vi "test Get-Set-Get Default Word Value.vi"(8 "error in":errorcluster, 11 "TestCase in":refnum<class "Scripting.lvclass">) -> (0 "error out":errorcluster, 3 "TestCase out":refnum<class "Scripting.lvclass">)   [LabVIEW 2020, in "Scripting.lvclass"]
uses:
  Scripting.lvclass
  Scripting.lvclass/Scripting.ctl
  <vilib>/addons/_JKI Toolkits/VI Tester/TestCase.llb/TestCase.lvclass
  Scripting/Ballard/Ballard ARINC 429 Scripting.lvlib
  Scripting/ARINC 429/ARINC 429 Scripting.lvlib
  C:/Program Files (x86)/National Instruments/LabVIEW 2020/vi.lib/addons/_JKI Toolkits/VI Tester/TestCase.llb/TestCase.lvclass
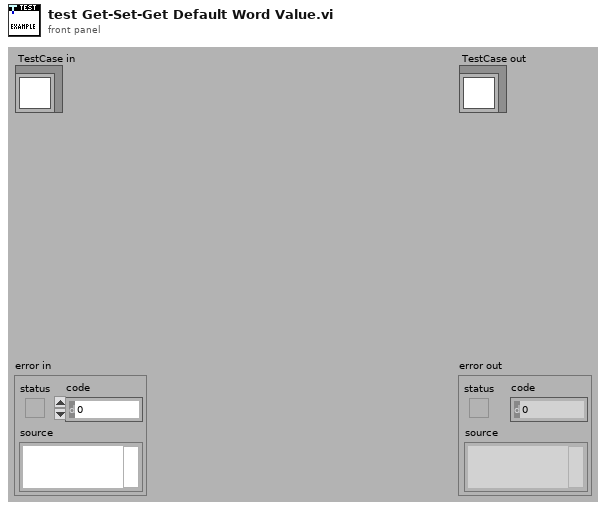
[diagram p1: front panel]
types:
  T1 = typedef "Custom Device API.lvlib/Custom Device Item Ref.ctl" = u64
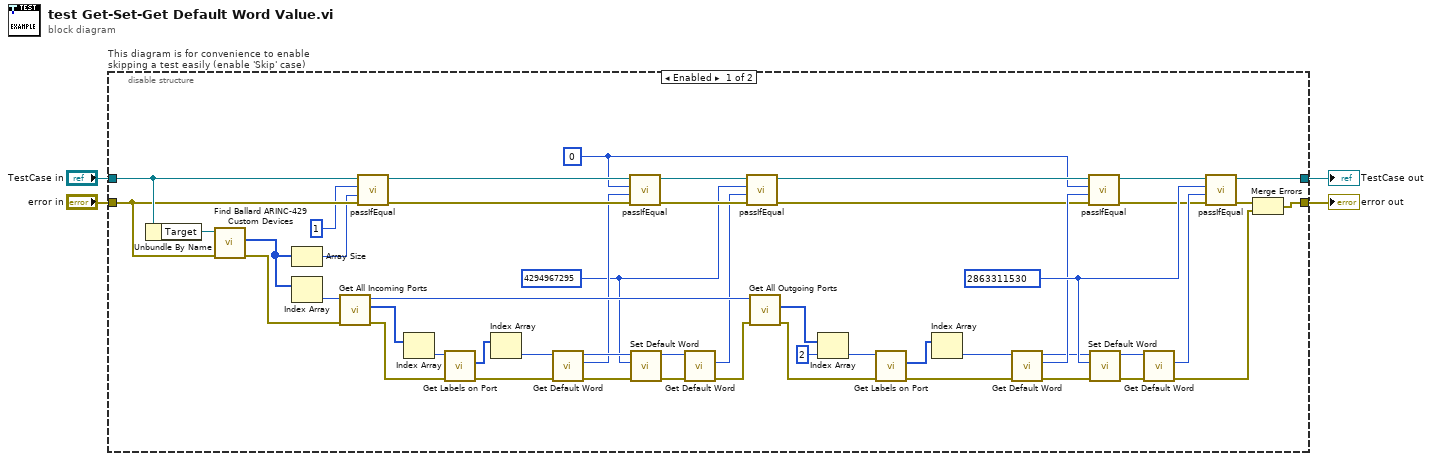
[diagram p0: block diagram]
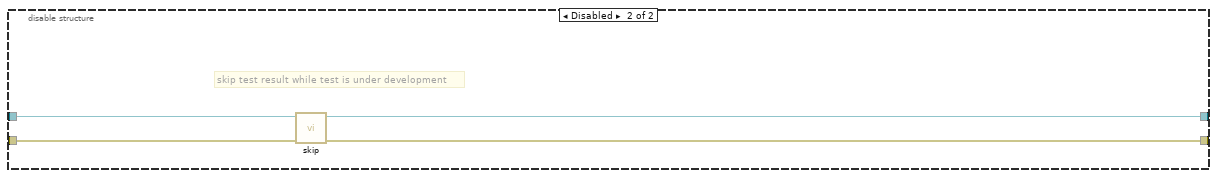
[diagram p2: hidden frame]
diagram:
  n1 = disable-structure "This diagram is for convenience to enable skipping a test easily (enable 'Skip' case)" shown="Enabled" {
    disable-tunnel: "TestCase in" -> [w52 w58]
    disable-tunnel: [w7 w56] -> w1
    disable-tunnel: [w43 w57] -> w3
    disable-tunnel: "error in" -> [w51 w55]
    frame Enabled {
      w21 = u32 2863311530 ("default word")
      w25 = u32 4294967295 ("default word")
      w6 = u32 0 ("default word")
      n2 = Unbundle By Name(w52) -> ("Target"=w54:refnum<k24>)
      n3 = call "Find Ballard ARINC-429 Custom Devices.vi"("error in"=w51, "target in"=w54) -> ("error out"=w47:errorcluster, "Ballard ARINC 429 custom devices"=w5:u64[])  [unwired: 7 in, 1 out]
      n4 = Array Size(array=w5) -> (size(s)=w49:i32)
      n5 = Index Array(array=w5) -> (element=w53:u64)  [unwired: 1 in]
      n6 = call "Get All Incoming Ports.vi"("error in"=w47, "Ballard ARINC 429 ref"=w53) -> ("error out"=w41:errorcluster, "Port refs"=w48:T1[], "Ballard ARINC 429 ref out"=w46:T1)  [unwired: 7 in]
      n7 = call-dynamic "passIfEqual.vi"("error in (no error)"=w51, "y"=w49, "x"=1 ("size(s)"), "TestCase in"=w52) -> ("error out"=w29:errorcluster, "TestCase out"=w30:refnum<class "Scripting.lvclass">)  [unwired: 6 in]
      n8 = Index Array(array=w48) -> (element=w42:T1)  [unwired: 1 in]
      n9 = call "Get Labels on Port.vi"("error in"=w41, "port ref"=w42) -> ("error out"=w36:errorcluster, "label references"=w37:T1[])  [unwired: 6 in, 2 out]
      n10 = Index Array(array=w37) -> (element=w35:T1)  [unwired: 1 in]
      n11 = call "Get Default Word.vi"("error in"=w36, "Item Ref in"=w35) -> ("error out"=w34:errorcluster, "default word"=w28:u32, "Item Ref out"=w33:T1)  [unwired: 7 in]
      n12 = call-dynamic "passIfEqual.vi"("error in (no error)"=w29, "y"=w28, "x"=w6, "TestCase in"=w30) -> ("error out"=w26:errorcluster, "TestCase out"=w27:refnum<class "Scripting.lvclass">)  [unwired: 6 in]
      n13 = call "Set Default Word.vi"("error in"=w34, "default word"=w25, "label ref in"=w33) -> ("error out"=w32:errorcluster, "label ref out"=w31:T1)  [unwired: 7 in]
      n14 = call "Get Default Word.vi"("error in"=w32, "Item Ref in"=w31) -> ("error out"=w23:errorcluster, "default word"=w24:u32)  [unwired: 7 in, 1 out]
      n15 = call-dynamic "passIfEqual.vi"("error in (no error)"=w26, "y"=w24, "x"=w25, "TestCase in"=w27) -> ("error out"=w14:errorcluster, "TestCase out"=w10:refnum<class "Scripting.lvclass">)  [unwired: 6 in]
      n16 = call "Get All Outgoing Ports.vi"("error in"=w23, "Ballard ARINC 429 ref"=w46) -> ("error out"=w40:errorcluster, "Port refs"=w45:T1[])  [unwired: 7 in, 1 out]
      n17 = Index Array(array=w45, index=2) -> (element=w39:T1)
      n18 = call "Get Labels on Port.vi"("error in"=w40, "port ref"=w39) -> ("error out"=w13:errorcluster, "label references"=w38:T1[])  [unwired: 6 in, 2 out]
      n19 = Index Array(array=w38) -> (element=w12:T1)  [unwired: 1 in]
      n20 = call "Get Default Word.vi"("error in"=w13, "Item Ref in"=w12) -> ("error out"=w15:errorcluster, "default word"=w19:u32, "Item Ref out"=w16:T1)  [unwired: 7 in]
      n21 = call-dynamic "passIfEqual.vi"("error in (no error)"=w14, "y"=w19, "x"=w6, "TestCase in"=w10) -> ("error out"=w20:errorcluster, "TestCase out"=w9:refnum<class "Scripting.lvclass">)  [unwired: 6 in]
      n22 = call "Set Default Word.vi"("error in"=w15, "default word"=w21, "label ref in"=w16) -> ("error out"=w17:errorcluster, "label ref out"=w18:T1)  [unwired: 7 in]
      n23 = call "Get Default Word.vi"("error in"=w17, "Item Ref in"=w18) -> ("error out"=w11:errorcluster, "default word"=w22:u32)  [unwired: 7 in, 1 out]
      n24 = call-dynamic "passIfEqual.vi"("error in (no error)"=w20, "y"=w22, "x"=w21, "TestCase in"=w9) -> ("error out"=w8:errorcluster, "TestCase out"=w7:refnum<class "Scripting.lvclass">)  [unwired: 6 in]
      n25 = Merge Errors(w8, w11) -> (w43:errorcluster)
    }
    frame Disabled {
      # "skip test result while test is under development"
      n26 = call <vilib>:"skip.vi"("error in (no error)"=w55, "TestCase in"=w58) -> ("error out"=w57:errorcluster, "TestCase out"=w56:refnum<class "Scripting.lvclass">)  [unwired: 8 in]
    }
  }
  "error out" <- w3
  "TestCase out" <- w1
